vi "checkData.vi"   [LabVIEW 2018]
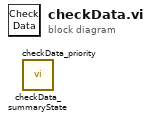
[diagram p0: block diagram]
diagram:
  n1 = call "checkData_summaryState.vi"() -> ()  [unwired: 10 in, 2 out]
  n2 = call "checkData_priority.vi"() -> ()  [unwired: 10 in, 2 out]
